vi "reglageSD.vi"(0 "Nombre d'acquisition par point (réglage)":u32) -> (1 "OD":cluster{"X":dbl[], "Y":dbl[]}, 2 "SC":T1(array[cluster]))   [LabVIEW 2015]
uses:
  globalVarSD.vi
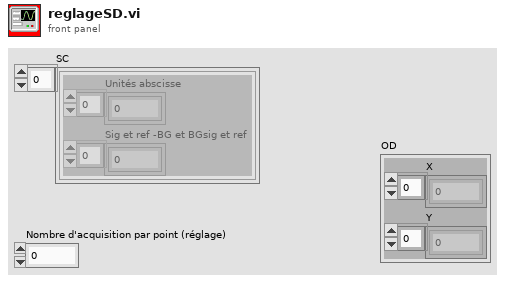
[diagram p1: front panel]
types:
  T1 = cluster{"Unités abscisse":dbl[], "Sig et ref -BG et BGsig et ref":dbl[]}[]
  T2 = cluster{"wavelengths":dbl[], "out array":dbl[]}[]
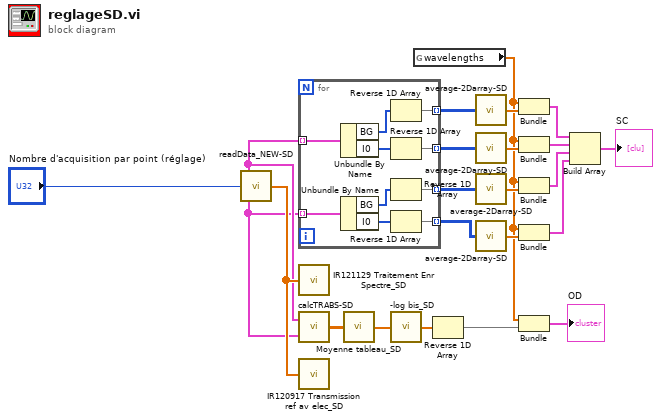
[diagram p0: block diagram]
diagram:
  n1 = call "readData_NEW-SD.vi"("how many points"="Nombre d'acquisition par point (réglage)") -> ("résultat début série"=w23:dbl[], "II channel seq"=w16:cluster{"BG":u16[], "Ie":u16[], "I0":u16[]}[], "I channel seq"=w17:cluster{"BG":u16[], "Ie":u16[], "I0":u16[]}[])
  n2 = for {
    tunnel: w17 -> [w33] mode=indexing
    tunnel: w16 -> [w30] mode=indexing
    tunnel: [w27] -> w15 mode=indexing
    tunnel: [w26] -> w14 mode=indexing
    tunnel: [w25] -> w13 mode=indexing
    tunnel: [w24] -> w12 mode=indexing
    n3 = Unbundle By Name(w33) -> ("BG"=w31:u16[], "I0"=w32:u16[])
    n4 = Unbundle By Name(w30) -> ("BG"=w29:u16[], "I0"=w28:u16[])
    n5 = Reverse 1D Array(array=w31) -> (reversed array=w27:u16[])
    n6 = Reverse 1D Array(array=w32) -> (reversed array=w26:u16[])
    n7 = Reverse 1D Array(array=w29) -> (reversed array=w25:u16[])
    n8 = Reverse 1D Array(array=w28) -> (reversed array=w24:u16[])
  }
  n9 = call "IR121129 Traitement Enr Spectre_SD.vi"("resultat_input"=w23) -> ()  [unwired: 1 out]
  n10 = call "calcTRABS-SD.vi"("II channel seq"=w16, "I channel seq"=w17) -> ("Résultat Transmission 2"=w18:dbl[][])
  n11 = call "IR120917 Transmission ref av elec_SD.vi"("resultat_input"=w23) -> ()  [unwired: 1 out]
  n12 = call "Moyenne tableau_SD.vi"("Signaux"=w18) -> ("Tableau"=w22:dbl[])
  n13 = call "-log bis_SD.vi"("Transmission"=w22) -> ("-log(x)=log(1/x)"=w20:dbl[])
  n14 = global read "globalVarSD.vi" "wavelengths"() -> (w1:dbl[])
  n15 = Reverse 1D Array(array=w20) -> (reversed array=w19:dbl[])
  n16 = call "average-2Darray-SD.vi"("2D array"=w15) -> ("out array"=w11:dbl[])
  n17 = call "average-2Darray-SD.vi"("2D array"=w14) -> ("out array"=w10:dbl[])
  n18 = call "average-2Darray-SD.vi"("2D array"=w13) -> ("out array"=w8:dbl[])
  n19 = call "average-2Darray-SD.vi"("2D array"=w12) -> ("out array"=w9:dbl[])
  n20 = Bundle("wavelengths"=w1, "out array"=w11) -> (w7:cluster{"wavelengths":dbl[], "out array":dbl[]})  [unwired: 1 in]
  n21 = Bundle("wavelengths"=w1, "out array"=w10) -> (w6:cluster{"wavelengths":dbl[], "out array":dbl[]})  [unwired: 1 in]
  n22 = Bundle("wavelengths"=w1, "out array"=w8) -> (w5:cluster{"wavelengths":dbl[], "out array":dbl[]})  [unwired: 1 in]
  n23 = Bundle("wavelengths"=w1, "out array"=w9) -> (w4:cluster{"wavelengths":dbl[], "out array":dbl[]})  [unwired: 1 in]
  n24 = Bundle("wavelengths"=w1, w19) -> (→"OD":cluster{"wavelengths":dbl[], dbl[]})  [unwired: 1 in]
  n25 = Build Array(w7, w6, w5, w4) -> (→"SC":T2)
